vi "Check time.vi"(9 "code":string) -> (3 "添加的路径":path)   [LabVIEW 2014]
panel:
  # "C:\\Database\\2022年9月30日"
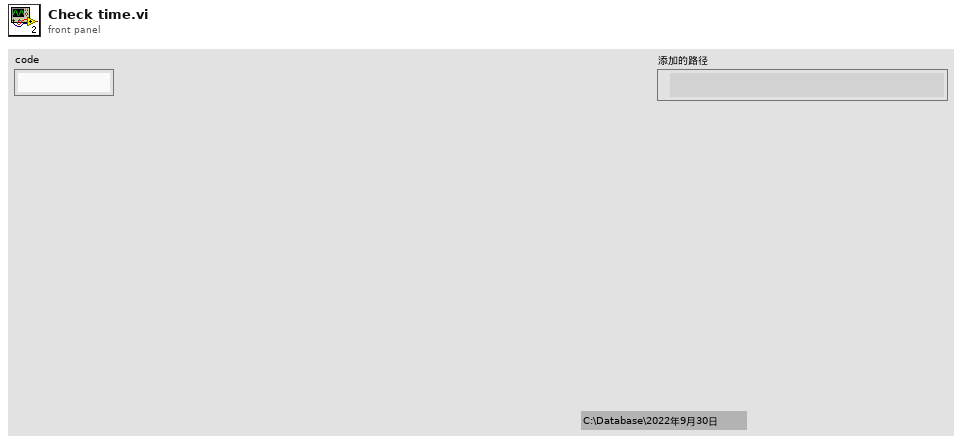
[diagram p1: front panel]
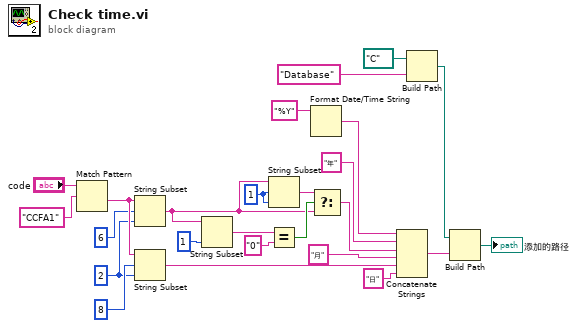
[diagram p0: block diagram]
diagram:
  w4 = 1 ("偏移量(0)")
  w16 = 2 ("长度（剩余）")
  n1 = Match Pattern(string="code", regular expression="CCFA1" ("正则表达式")) -> (after substring=w19:string)  [unwired: 1 in, 3 out]
  n2 = String Subset(string=w19, offset (0)=6 ("偏移量(0)"), length (rest)=w16) -> (substring=w2:string)
  n3 = String Subset(string=w19, offset (0)=8 ("偏移量(0)"), length (rest)=w16) -> (substring=w17:string)
  n4 = String Subset(string=w2, length (rest)=1 ("长度（剩余）")) -> (substring=w7:string)  [unwired: 1 in]
  n5 = String Subset(string=w2, offset (0)=w4, length (rest)=w4) -> (substring=w3:string)
  n6 = Equal?(x=w7, y="0") -> (x = y?=w5:bool)
  n7 = Format Date/Time String(time format string (%c)="%Y" ("时间格式字符串(%c)")) -> (date/time string=w9:string)  [unwired: 2 in]
  n8 = Select(t=w3, s=w5, f=w2) -> (s? t:f=w1:string)
  n9 = Concatenate Strings(w9, "年" ("字符串"), w1, "月" ("字符串"), w17, "日" ("字符串")) -> (w22:string)
  n10 = Build Path(base path=path "C:/" ("path"), name or relative path="Database" ("file name")) -> (appended path=w11:path)
  n11 = Build Path(base path=w11, name or relative path=w22) -> (appended path=→"添加的路径":path)
